vi "PH_SSAC.set GUI Elements.vi"(0 "i ref in":refnum<vi>, 5 "error in":errorcluster) -> (14 "i ref out":refnum<vi>, 19 "error out":errorcluster)   [LabVIEW 2014, in "PH_SSAC.lvlib"]
uses:
  PH_SSAC.lvlib
  PH_Basics/PH_Common/PH_Common.lvlib
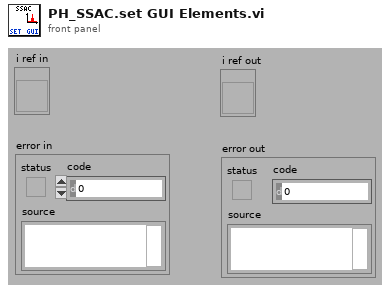
[diagram p1: front panel]
types:
  T1 = typedef "PH_SSAC.lvlib/PH_SSAC.i attribute.ctl" = cluster{"GUI Refs":cluster{"Delete":refnum<vi>, "Global On":refnum<vi>, "Cam Source":refnum<vi>, "Frame Main Signal":refnum<vi>, "Frame Background":refnum<vi>, "dt (Gauss smooth)":refnum<vi>, "Calibration Factor":refnum<vi>, "Background acquire":refnum<vi>, "Threshold":refnum<vi>, "Time evolution of mean pulse duration":refnum<vi>, "Mean Pulse Duration":refnum<vi>, "Main signal":refnum<vi>, "Current Pulse Duration":refnum<vi>, "Processed":refnum<vi>, "Saturation":refnum<vi>, "# for Average":refnum<vi>, "Position":refnum<vi>, "BG Status":refnum<vi>, "Save BG data":refnum<vi>, "Read BG Data":refnum<vi>, "Background Calibration Data":refnum<vi>}, "Images":cluster{"OP Image":T2, "GUI Image":T2, "PSDB Image":T2}, "Global On?":bool, "Frame Main":cluster{"x":u32, "dx":u32, "y":u32, "dy":u32}, "Frame Background":cluster{"x":u32, "dx":u32, "y":u32, "dy":u32}, "dt [fs]":dbl, "Calibration Factor [fs/pixel]":dbl, "Threshold":dbl, "Time evolution of mean pulse duration [fs]":dbl[], "Main Signal":cluster{"Time for Main":dbl[], "Signal":dbl[]}, "Processed":bool, "Current Pulse Duration [fs]":dbl, "# for Average":i32, "Position":i32, "Pulse Durations [fs]":dbl[], "BG":cluster{"Acquire?":bool, "Background Calibration Data":T3, "Save Data":bool}}
  T2 = typedef "IMAQ Image.ctl" = refnum<image>
  T3 = typedef "PH_SSAC.lvlib/PH_SSAC.Background Data.ctl" = cluster{"Date":string, "Time":string, "Frame Main":cluster{"x":u32, "dx":u32, "y":u32, "dy":u32}, "dt [fs]":dbl, "Calibration Factor [fs/pixel]":dbl, "Signal":dbl[], "Frame Background":cluster{"x":u32, "dx":u32, "y":u32, "dy":u32}}
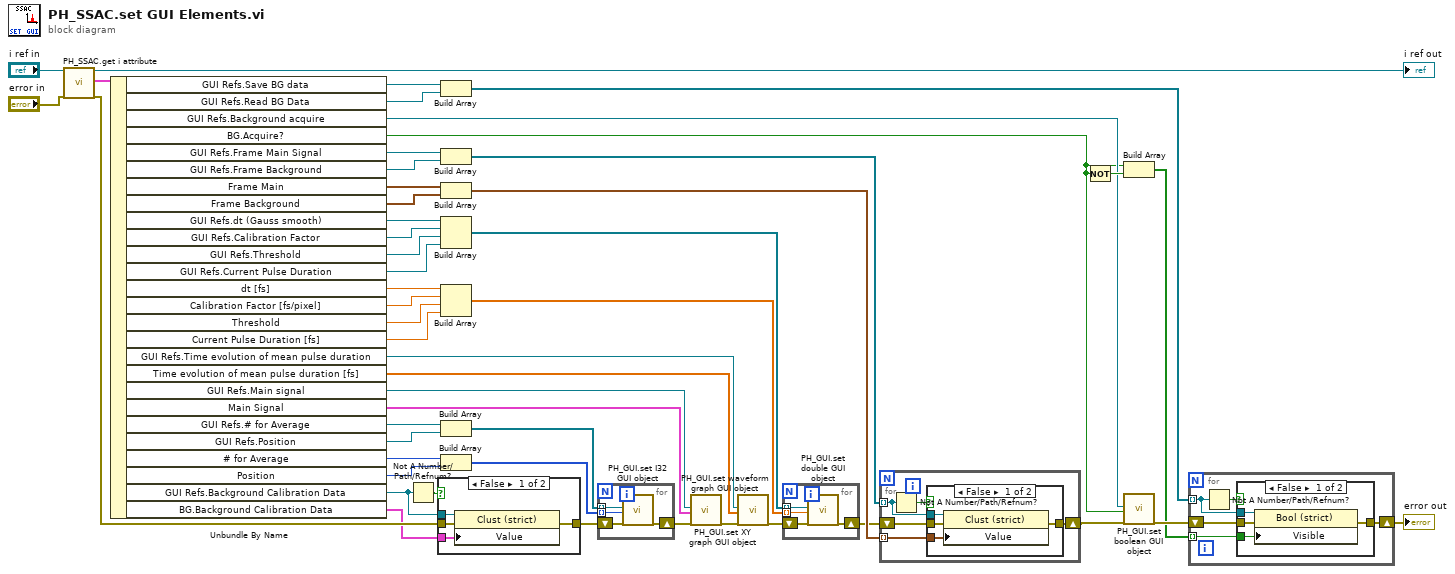
[diagram p0: block diagram]
diagram:
  n1 = call "PH_SSAC.get i attribute.vi"("i ref in"="i ref in", "error in (no error)"="error in") -> ("i ref out"=→"i ref out":refnum<vi>, "i attribute"=w46:T1, "error out"=w49:errorcluster)  [unwired: 15 in]
  n2 = Unbundle By Name(w46) -> ("GUI Refs.Save BG data"=w11:refnum<vi>, "GUI Refs.Read BG Data"=w10:refnum<vi>, "GUI Refs.Background acquire"=w6:refnum<vi>, "BG.Acquire?"=w5:bool, "GUI Refs.Frame Main Signal"=w17:refnum<vi>, "GUI Refs.Frame Background"=w16:refnum<vi>, "Frame Main"=w45:cluster{"x":u32, "dx":u32, "y":u32, "dy":u32}, "Frame Background"=w44:cluster{"x":u32, "dx":u32, "y":u32, "dy":u32}, "GUI Refs.dt (Gauss smooth)"=w43:refnum<vi>, "GUI Refs.Calibration Factor"=w42:refnum<vi>, "GUI Refs.Threshold"=w41:refnum<vi>, "GUI Refs.Current Pulse Duration"=w40:refnum<vi>, "dt [fs]"=w38:dbl, "Calibration Factor [fs/pixel]"=w37:dbl, "Threshold"=w36:dbl, "Current Pulse Duration [fs]"=w35:dbl, "GUI Refs.Time evolution of mean pulse duration"=w32:refnum<vi>, "Time evolution of mean pulse duration [fs]"=w31:dbl[], "GUI Refs.Main signal"=w29:refnum<vi>, "Main Signal"=w30:cluster{"Time for Main":dbl[], "Signal":dbl[]}, "GUI Refs.# for Average"=w27:refnum<vi>, "GUI Refs.Position"=w26:refnum<vi>, "# for Average"=w24:i32, "Position"=w23:i32, "GUI Refs.Background Calibration Data"=w19:refnum<vi>, "BG.Background Calibration Data"=w18:T3)
  n3 = Not A Number/Path/Refnum?(number/path/refnum=w19) -> (NaN/Path/Refnum?=w20:bool)
  n4 = case shown="False" w20 {
    tunnel: w49 -> [w53 w54]
    tunnel: [w52 w54] -> w21
    tunnel: w19 -> [w51 _]
    tunnel: w18 -> [w50 _]
    frame False {
      n5 = property class="Clust (strict)"(reference=w51, error in=w53, "Value"=w50) -> (error out=w52:errorcluster)  [unwired: 1 out]
    }
    frame True {
    }
  }
  n6 = Build Array(w11, w10) -> (w9:refnum<vi>[])
  n7 = Build Array(w17, w16) -> (w15:refnum<vi>[])
  n8 = Build Array(w45, w44) -> (w14:cluster{"x":u32, "dx":u32, "y":u32, "dy":u32}[])
  n9 = Build Array(w43, w42, w41, w40) -> (w39:refnum<vi>[])
  n10 = Build Array(w38, w37, w36, w35) -> (w34:dbl[])
  n11 = Build Array(w27, w26) -> (w25:refnum<vi>[])
  n12 = Build Array(w24, w23) -> (w22:i32[])
  n13 = for {
    shift-right: [w57] -> w28
    shift-left: w21 -> [w58]
    tunnel: w25 -> [w56] mode=indexing
    tunnel: w22 -> [w55] mode=indexing
    n14 = call "PH_GUI.set I32 GUI object.vi"("I32 GUI Ref"=w56, "value"=w55, "error in (no error)"=w58) -> ("error out"=w57:errorcluster)  [unwired: 16 in]
  }
  n15 = call "PH_GUI.set XY graph GUI object.vi"("XY Graph GUI Ref"=w29, "Value Cluster"=w30, "error in"=w28) -> ("error out"=w4:errorcluster)  [unwired: 16 in]
  n16 = call "PH_GUI.set waveform graph GUI object.vi"("Graph GUI Ref"=w32, "Values"=w31, "error in"=w4) -> ("error out"=w33:errorcluster)  [unwired: 16 in]
  n17 = for {
    shift-right: [w61] -> w3
    shift-left: w33 -> [w62]
    tunnel: w39 -> [w60] mode=indexing
    tunnel: w34 -> [w59] mode=indexing
    n18 = call "PH_GUI.set double GUI object.vi"("GUI object Ref"=w60, "value"=w59, "error in (no error)"=w62) -> ("error out"=w61:errorcluster)  [unwired: 16 in]
  }
  n19 = for {
    shift-right: [w67] -> w8
    shift-left: w3 -> [w66]
    tunnel: w15 -> [w64] mode=indexing
    tunnel: w14 -> [w63] mode=indexing
    n20 = Not A Number/Path/Refnum?(number/path/refnum=w64) -> (NaN/Path/Refnum?=w65:bool)
    n21 = case shown="False" w65 {
      tunnel: w66 -> [w71 w72]
      tunnel: [w70 w72] -> w67
      tunnel: w64 -> [w69 _]
      tunnel: w63 -> [w68 _]
      frame False {
        n22 = property class="Clust (strict)"(reference=w69, error in=w71, "Value"=w68) -> (error out=w70:errorcluster)  [unwired: 1 out]
      }
      frame True {
      }
    }
  }
  n23 = Not(x=w5) -> (.not. x?=w13:bool)
  n24 = Build Array(w5, w13) -> (w7:bool[])
  n25 = call "PH_GUI.set boolean GUI object.vi"("Boolean Knob GUI Ref"=w6, "Value"=w5, "error in (no error)"=w8) -> ("error out"=w12:errorcluster)  [unwired: 16 in]
  n26 = for {
    shift-right: [w76] -> w47
    shift-left: w12 -> [w77]
    tunnel: w9 -> [w75] mode=indexing
    tunnel: w7 -> [w73] mode=indexing
    n27 = Not A Number/Path/Refnum?(number/path/refnum=w75) -> (NaN/Path/Refnum?=w74:bool)
    n28 = case shown="False" w74 {
      tunnel: w77 -> [w81 w82]
      tunnel: [w80 w82] -> w76
      tunnel: w75 -> [w79 _]
      tunnel: w73 -> [w78 _]
      frame False {
        n29 = property class="Bool (strict)"(reference=w79, error in=w81, "Visible"=w78) -> (error out=w80:errorcluster)  [unwired: 1 out]
      }
      frame True {
      }
    }
  }
  "error out" <- w47
